vi "2-4.vi"() -> ()   [LabVIEW 2018]
uses:
  <vilib>/Analysis/3filter.llb/Filter Passband Type.ctl
  <vilib>/Analysis/3filter.llb/Butterworth Filter (DBL).vi
  <vilib>/express/express analysis/Spectral/Block/exnSpectralBlock spectral measurements peak poly.vi
  <vilib>/express/express analysis/Spectral/Block/exnSpectralBlock spectral measurements peak WFM.vi
  <vilib>/express/express analysis/Spectral/XNode/ExpressSpectralMeasurementsBlockNode.xnode
  <vilib>/measure/NI_MABase.lvlib
  <vilib>/Analysis/NI_AALPro.lvlib
  <vilib>/Analysis/NI_AALBase.lvlib
  <vilib>/measure/NI_MAPro.lvlib
panel:
  in  "停止":bool
  in  "带通Butterworth滤波器":cluster{"中心频率(Hz)":dbl, "带宽(Hz)":dbl}={"中心频率(Hz)"=150000.0, "带宽(Hz)"=220000.0}
  out "fh":dbl
  out "fl":dbl
  in  "选项卡控件":enum32{"调制", "滤波", "解调"}(tab)
  out "频域":cluster{"f0":dbl, "df":dbl, "magnitude":dbl[]}(graph)
  out "时域":waveform(dbl)[](graph)
  out "频域":cluster{"f0":dbl, "df":dbl, "magnitude":dbl[]}(graph)
  out "时域":waveform(dbl)(graph)
  out "时域 2":waveform(dbl)[](graph)
  out "BT(Hz)":dbl
  out "数组":dbl[](array[numeric])
  out "调制信号":waveform(dbl)(graph)
  out "积分信号":waveform(dbl)(graph)
  out "采样参数（采样频率fs，采样数Ns）":cluster{dbl, dbl} {"?" format="%#_6f"; "?" format="%#_6f"}
  out "载波信号":waveform(dbl)(graph)
  in  "kf(Hz/V)":dbl=50000.0
  in  "An(V)":dbl=0.1
  in  "调制信号":cluster{"T(s)":dbl, "Am(V)":dbl}={"T(s)"=0.0002, "Am(V)"=1.0}
  in  "载波信号":cluster{"fc(Hz)":dbl, "Ac(V)":dbl}={"fc(Hz)"=150000.0, "Ac(V)"=1.0}
  # "要显示n个周期的调制信号波形，\n则采样数Ns=n*fs/fm\n为了减小运算量这里仅使用\n100*fc作为采样频率"
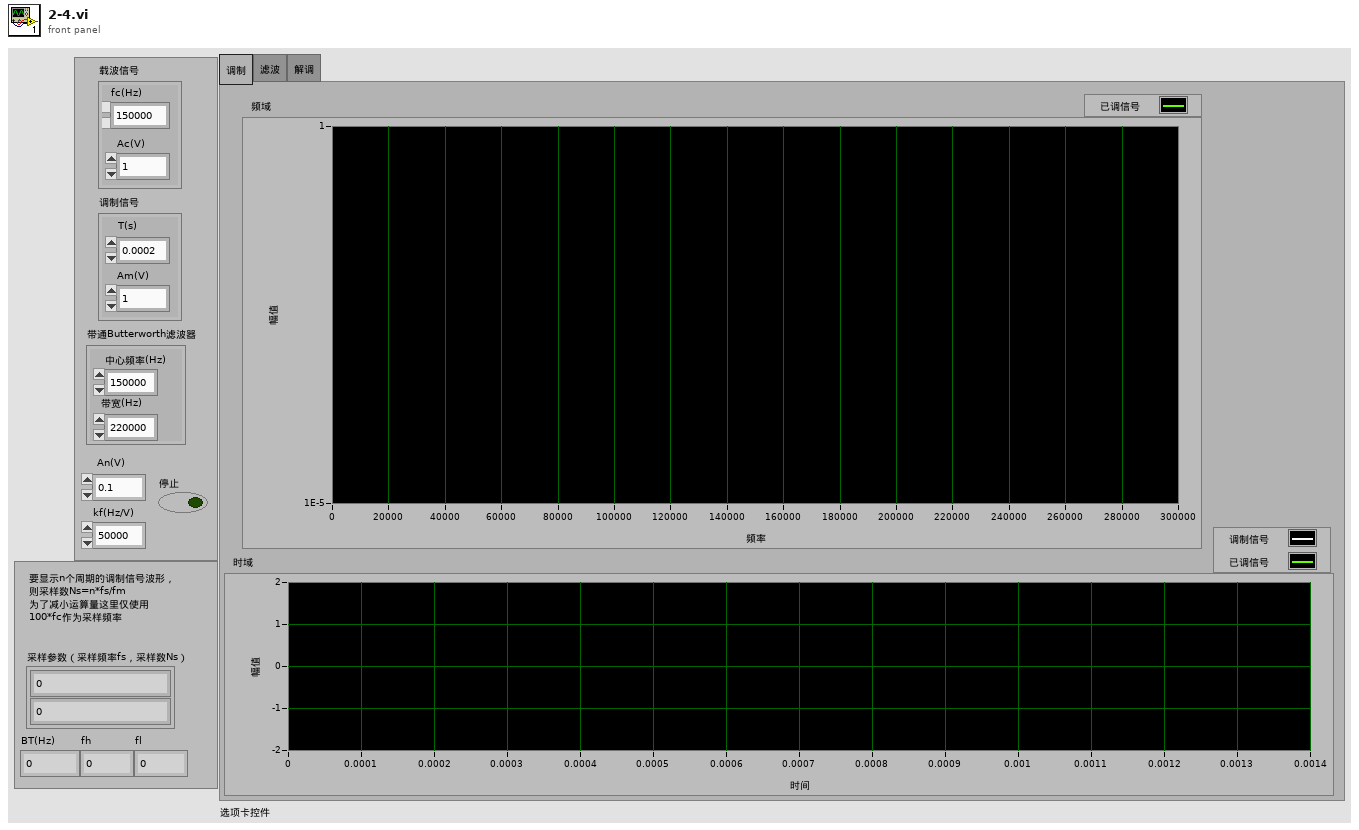
[diagram p1: front panel]
types:
  T1 = typedef "NI_AALBase.lvlib/Filter Passband Type.ctl" = enum32{"Lowpass", "Highpass", "Bandpass", "Bandstop"}
  T2 = cluster{"averaging mode":u16, "weighting mode":u16, "number of averages":u32}
  T3 = cluster{"dB On (F)":bool, "unwrap phase (F)":bool, "convert to degree (F)":bool}
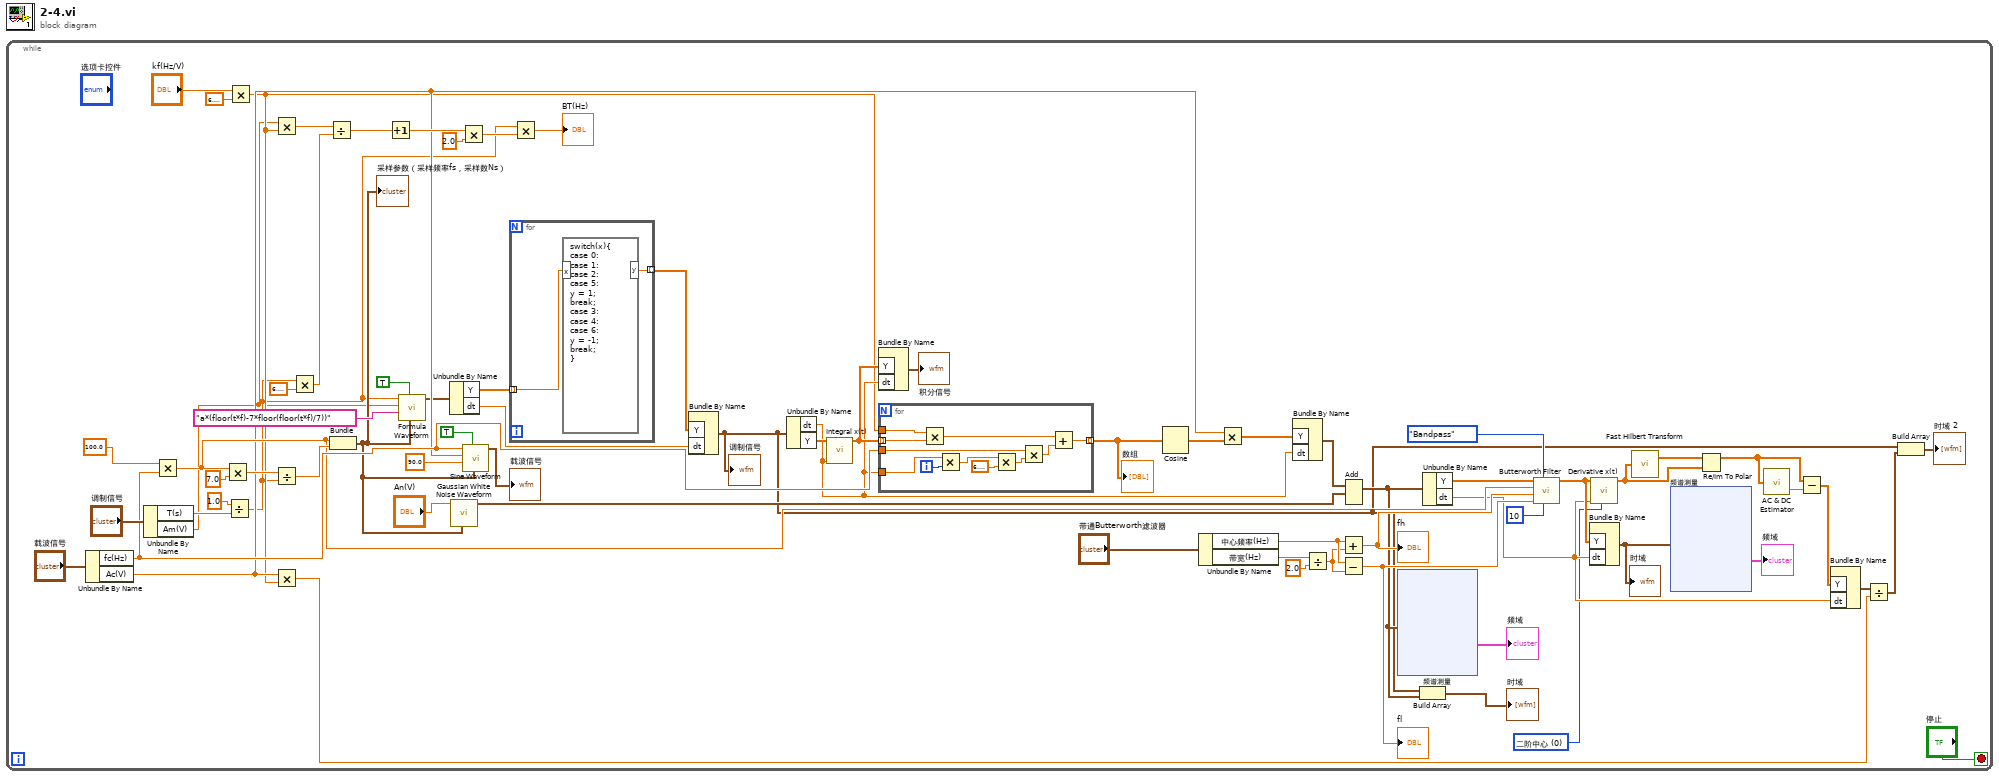
[diagram p0: block diagram]
diagram:
  n1 = while {
    stop <- "停止" stop-if-true
    w26 = u16 0 items=["二阶中心", "四阶中心", "前向", "后向"] ("method")
    n2 = Unbundle By Name("载波信号") -> ("fc(Hz)"=w62:dbl, "Ac(V)"=w22:dbl)
    n3 = Unbundle By Name("调制信号") -> ("T(s)"=w12:dbl, "Am(V)"=w2:dbl)
    n4 = Multiply(x=100.0, y=w62) -> (x*y=w34:dbl)
    n5 = Multiply(x=w34, y=7.0) -> (x*y=w68:dbl)
    n6 = Divide(x=1.0, y=w12) -> (x/y=w9:dbl)
    n7 = Multiply(x="kf(Hz/V)", y=6.283185307179586) -> (x*y=w16:dbl)
    n8 = Multiply(x=w2, y=w16) -> (x*y=w49:dbl)
    n9 = Divide(x=w68, y=w9) -> (x/y=w67:dbl)
    n10 = Multiply(x=w22, y=w16) -> (x*y=w20:dbl)
    n11 = Multiply(x=w9, y=6.283185307179586) -> (x*y=w50:dbl)
    n12 = Divide(x=w49, y=w50) -> (x/y=w48:dbl)
    n13 = Bundle(w34, w67) -> (w10:cluster{dbl, dbl})  [unwired: 1 in]
    "采样参数（采样频率fs，采样数Ns）" <- w10
    n14 = Increment(x=w48) -> (x+1=w47:dbl)
    n15 = call <vilib>:"Formula Waveform.vi"("sampling info"=w10, "reset signal"=TRUE, "formula"="a*(floor(t*f)-7*floor(floor(t*f)/7))", "amplitude"=w2, "frequency"=w9) -> ("signal out"=w8:waveform(dbl))  [unwired: 5 in, 1 out]
    n16 = Unbundle By Name(w8) -> ("Y"=w6:dbl[], "dt"=w7:dbl)
    n17 = call <vilib>:"Gaussian White Noise Waveform.vi"("sampling info"=w10, "standard deviation"="An(V)") -> ("signal out"=w54:waveform(dbl))  [unwired: 8 in, 1 out]
    n18 = Multiply(x=w47, y=2.0) -> (x*y=w45:dbl)
    n19 = call <vilib>:"Sine Waveform.vi"("sampling info"=w10, "reset signal"=TRUE, "phase"=90.0, "amplitude"=w22, "frequency"=w62) -> ("signal out"=→"载波信号":waveform(dbl))  [unwired: 5 in, 1 out]
    n20 = for {
      tunnel: w6 -> [w75] mode=indexing
      tunnel: [w74] -> w5 mode=indexing
      n21 = formula code="switch(x){\ncase 0:\ncase 1:\ncase 2:\ncase 5:\ny = 1;\nbreak;\ncase 3:\ncase 4:\ncase 6:\ny = -1;\nbreak;\n}"("x"=w75) -> ("y"=w74:dbl)
    }
    n22 = Multiply(x=w9, y=w45) -> (x*y=→"BT(Hz)":dbl)
    n23 = Bundle By Name("Y"=w5, "dt"=w7) -> (w3:waveform(dbl))  [unwired: 1 in]
    "调制信号" <- w3
    n24 = Unbundle By Name(w3) -> ("dt"=w59:dbl, "Y"=w69:dbl[])
    n25 = call <vilib>:"Integral x(t).vi"("dt"=w59, "X"=w69) -> ("Integral X"=w63:dbl[])  [unwired: 8 in, 1 out]
    n26 = Bundle By Name("Y"=w63, "dt"=w59) -> (→"积分信号":waveform(dbl))  [unwired: 1 in]
    n27 = for {
      tunnel: w63 -> [w106] mode=indexing
      tunnel: w59 -> [w104]
      tunnel: w62 -> [w100]
      tunnel: [w97] -> w61 mode=indexing
      tunnel: w16 -> [w96]
      i -> [w105]
      n28 = Multiply(x=w96, y=w106) -> (x*y=w98:dbl)
      n29 = Multiply(x=w104, y=w105) -> (x*y=w102:dbl)
      n30 = Multiply(x=w102, y=6.283185307179586) -> (x*y=w101:dbl)
      n31 = Multiply(x=w100, y=w101) -> (x*y=w99:dbl)
      n32 = Add(x=w98, y=w99) -> (x+y=w97:dbl)
    }
    "数组" <- w61
    n33 = Cosine(x=w61) -> (cos(x)=w60:dbl[])
    n34 = Unbundle By Name("带通Butterworth滤波器") -> ("中心频率(Hz)"=w36:dbl, "带宽(Hz)"=w40:dbl)
    n35 = Multiply(x=w22, y=w60) -> (x*y=w58:dbl[])
    n36 = Bundle By Name("Y"=w58, "dt"=w59) -> (w56:waveform(dbl))  [unwired: 1 in]
    n37 = Divide(x=w40, y=2.0) -> (x/y=w35:dbl)
    n38 = Add(1:w54, 2:w56) -> (0:w32:waveform(dbl))  [unwired: 1 in, 1 out]
    n39 = Add(x=w36, y=w35) -> (x+y=w38:dbl)
    "fh" <- w38
    n40 = Subtract(x=w36, y=w35) -> (x-y=w37:dbl)
    "fl" <- w37
    n41 = xnode "频谱测量"("信号"=w32) -> ("FFT - （峰值）"=→"频域":cluster{"f0":dbl, "df":dbl, "magnitude":dbl[]})  [unwired: 1 in, 2 out]
    n42 = Build Array(w3, w32) -> (→"时域":waveform(dbl)[])
    n43 = Unbundle By Name(w32) -> ("Y"=w31:dbl[], "dt"=w27:dbl)
    n44 = call-poly <vilib>:"Butterworth Filter.vi"("order"=10, "filter type"=Filter_Passband_Type."Bandpass", "low cutoff freq: fl"=w37, "high cutoff freq: fh"=w38, "sampling freq: fs"=w34, "X"=w31) -> ("Filtered X"=w29:dbl[])  [unwired: 2 in, 1 out]
    n45 = Bundle By Name("Y"=w29, "dt"=w27) -> (w30:waveform(dbl))  [unwired: 1 in]
    "时域" <- w30
    n46 = call <vilib>:"Derivative x(t).vi"("method"=w26, "dt"=w27, "X"=w29) -> ("dX/dt"=w19:dbl[])  [unwired: 7 in, 1 out]
    n47 = call <vilib>:"Fast Hilbert Transform.vi"("X"=w19) -> ("Hilbert{X}"=w28:dbl[])  [unwired: 1 out]
    n48 = xnode "频谱测量"("信号"=w30) -> ("FFT - （峰值）"=→"频域":cluster{"f0":dbl, "df":dbl, "magnitude":dbl[]})  [unwired: 1 in, 2 out]
    n49 = Re/Im To Polar(2:w19, 3:w28) -> (1:w25:dbl[])  [unwired: 1 out]
    n50 = call <vilib>:"AC & DC Estimator.vi"("Signal (V)"=w25) -> ("DC estimate (V)"=w24:dbl)  [unwired: 1 out]
    n51 = Subtract(x=w25, y=w24) -> (x-y=w23:dbl[])
    n52 = Bundle By Name("Y"=w23, "dt"=w27) -> (w21:waveform(dbl))  [unwired: 1 in]
    n53 = Divide(x=w21, y=w20) -> (x/y=w15:waveform(dbl))
    n54 = Build Array(w3, w15) -> (→"时域 2":waveform(dbl)[])
  }
